vi "Index.vi"(10 "Shoot":bool, 11 "Output 2":dbl=-0.007874015748031496 format="%#_13g") -> ()   [LabVIEW 2016]
panel:
  in  "Output":dbl=-0.007874015748031496 format="%#_13g"
  in  "Max Effort":dbl=0.5 format="%#_13g"
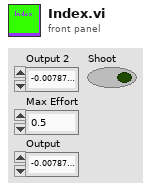
[diagram p1: front panel]
types:
  T1 = typedef "WPI_MotorControlDeviceRef.ctl" = cluster{"DeviceStatus":errorcluster, "Type":T2, "PWM":cluster{"PWM Channel":T3, "DeadBand":T4}, "CAN":cluster{"Device Number":u8, "SetOutput VI Ref":variant, "GetOutput VI Ref":variant, "Enable VI Ref":variant, "Disable VI Ref":variant, "Data":variant}, "Invert":bool}
  T2 = typedef "WPI_MotorControlType.ctl" = enum16{"PWM", "CAN"}
  T3 = typedef "FPGA_DIOPWMChannel.ctl" = enum8{"PWM 0", "PWM 1", "PWM 2", "PWM 3", "PWM 4", "PWM 5", "PWM 6", "PWM 7", "PWM 8", "PWM 9", "PWM MXP 0", "PWM MXP 1", "PWM MXP 2", "PWM MXP 3", "PWM MXP 4", "PWM MXP 5", "PWM MXP 6", "PWM MXP 7", "PWM MXP 8", "PWM MXP 9", "Invalid"}
  T4 = typedef "WPI_PWMDeadband.ctl" = cluster{"Name":string, "maxPositivePwm":i32, "minPositivePwm":i32, "centerPwm":i32, "maxNegativePwm":i32, "minNegativePwm":i32, "angularRange":u16}
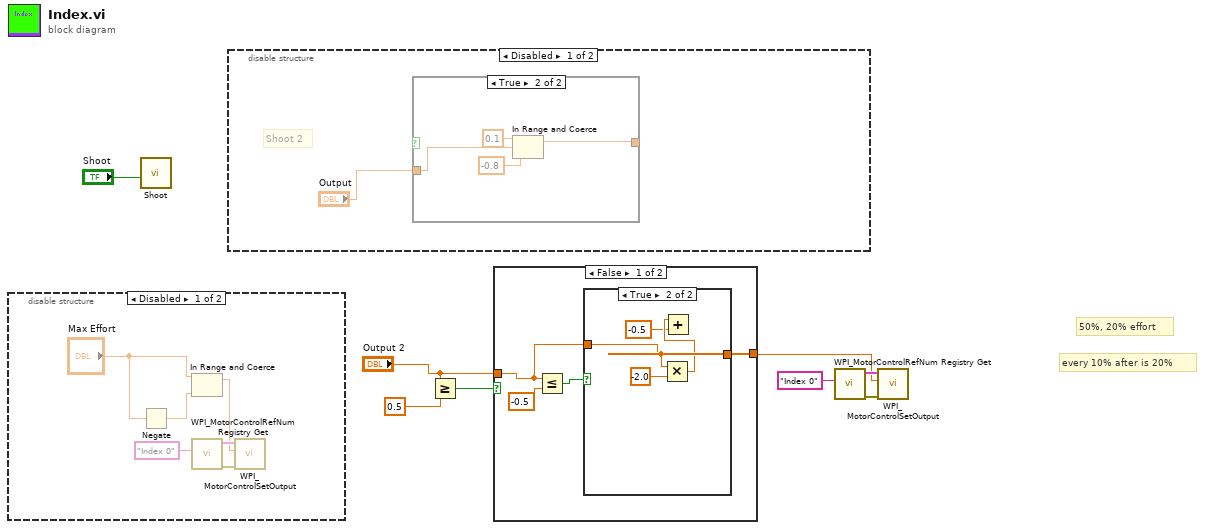
[diagram p0: block diagram]
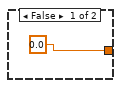
[diagram p2: hidden frame]
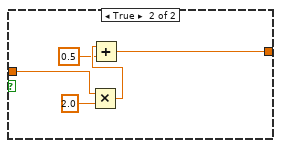
[diagram p3: hidden frame]
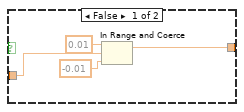
[diagram p4: hidden frame]
diagram:
  # "50%, 20% effort"
  # "every 10% after is 20%"
  n1 = disable-structure shown="Disabled" {
    frame Disabled {
      n2 = Negate(x="Max Effort") -> (-x=w10:dbl)
      n3 = In Range and Coerce(upper limit="Max Effort", lower limit=w10) -> (coerced(x)=w11:dbl)  [unwired: 1 in, 1 out]
      n4 = call <vilib>:"WPI_MotorControlRefNum Registry Get.vi"("refnum name"="Index 0") -> ("error out"=w13:errorcluster, "MotorControlDevRef"=w14:T1)  [unwired: 9 in]
      n5 = call <vilib>:"WPI_MotorControlSetOutput.vi"("error in (no error)"=w13, "Output"=w11, "MotorControlDevRef"=w14) -> ()  [unwired: 6 in, 3 out]
    }
    frame Enabled {
    }
  }
  n6 = call "Shoot.vi"("Shoot"="Shoot") -> ()  [unwired: 10 in]
  n7 = disable-structure shown="Disabled" {
    frame Disabled {
      # "Shoot 2"
      n8 = case shown="True" w16 {
        tunnel: "Output" -> [w20 w24]
        tunnel: [w17 w21] -> _
        frame False {
          n9 = In Range and Coerce(upper limit=0.01, x=w20, lower limit=-0.01 ("upper limit")) -> (coerced(x)=w17:dbl)  [unwired: 1 out]
        }
        frame True {
          n10 = In Range and Coerce(upper limit=0.1, x=w24, lower limit=-0.8 ("upper limit")) -> (coerced(x)=w21:dbl)  [unwired: 1 out]
        }
      }
    }
    frame Enabled {
    }
  }
  n11 = Greater Or Equal?(x="Output 2", y=0.5) -> (x >= y?=w6:bool)
  n12 = case shown="False" w6 {
    tunnel: "Output 2" -> [w26 w38]
    tunnel: [w25 w34] -> w1
    frame False {
      n13 = Less Or Equal?(x=w26, y=-0.5) -> (x <= y?=w28:bool)
      n14 = case shown="True" w28 {
        tunnel: w26 -> [_ w30]
        tunnel: [0.0 w30] -> w25
        frame False {
        }
        frame True {
          n15 = Multiply(x=w30, y=-2.0) -> (x*y=w32:dbl)
          n16 = Add(x=w32, y=-0.5) -> ()  [unwired: 1 out]
        }
      }
    }
    frame True {
      n17 = Multiply(x=w38, y=2.0) -> (x*y=w36:dbl)
      n18 = Add(x=w36, y=0.5) -> (x+y=w34:dbl)
    }
  }
  n19 = call <vilib>:"WPI_MotorControlRefNum Registry Get.vi"("refnum name"="Index 0") -> ("error out"=w3:errorcluster, "MotorControlDevRef"=w2:T1)  [unwired: 9 in]
  n20 = call <vilib>:"WPI_MotorControlSetOutput.vi"("error in (no error)"=w3, "Output"=w1, "MotorControlDevRef"=w2) -> ()  [unwired: 6 in, 3 out]
